vi "Keysight 34461A Measurement Logic.vi"(8 "error in (no error)":errorcluster, 10 "session":refnum<visa-resource-name>, 11 "measurement configuration":T2={"pin_name"="", "measurement_type"=enum."DC Voltage", "auto_range"=FALSE, "manual_range"=0.0, "resolution_digits"=0.0}) -> (0 "error out":errorcluster, 3 "measurement results":T1)   [LabVIEW 2021, in "Keysight 34461A DMM Measurement.lvlib"]
uses:
  Keysight 34461A DMM Measurement.lvlib
  Measurement Results.ctl
  <instrlib>/Agilent 3446X Series/Agilent 3446X Series.lvlib
  <instrlib>/Agilent 3446X Series/Public/Data/Read (Single Point).vi
  Measurement Configuration.ctl
  Keysight 34461A Function.ctl
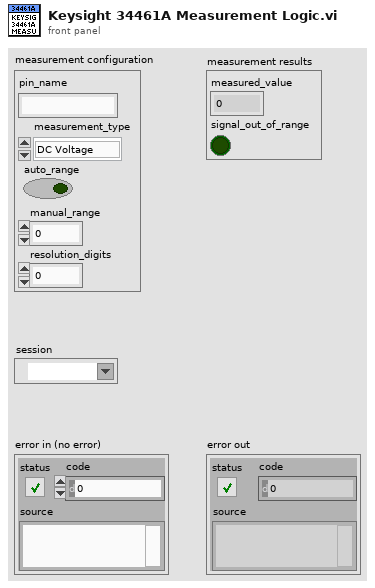
[diagram p1: front panel]
types:
  T1 = typedef "Keysight 34461A DMM Measurement.lvlib/Measurement Results.ctl" = cluster{"measured_value":dbl, "signal_out_of_range":bool}
  T2 = typedef "Keysight 34461A DMM Measurement.lvlib/Measurement Configuration.ctl" = cluster{"pin_name":string, "measurement_type":T3, "auto_range":bool, "manual_range":dbl, "resolution_digits":dbl}
  T3 = typedef "Keysight 34461A DMM Measurement.lvlib/Keysight 34461A Function.ctl" = enum32{"Continuity", "AC Current", "DC Current", "Diode Checking", "Frequency", "4 - Wire Resistance", "Period", "2 - Wire Resistance", "Temperature", "AC Voltage", "DC Voltage", "VDC:VDC Ratio", "Capacitance"}
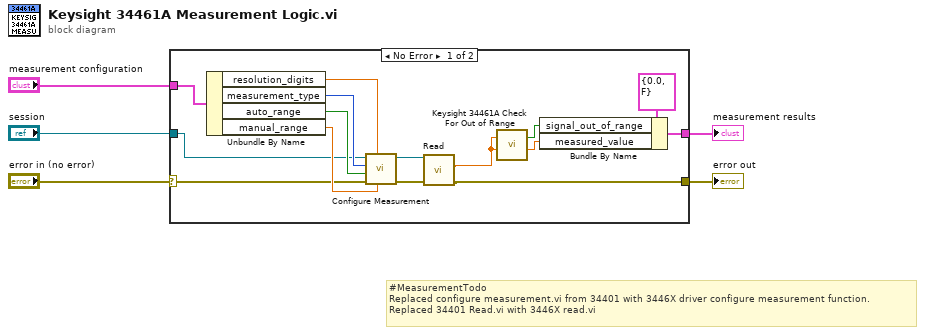
[diagram p0: block diagram]
diagram:
  # "#MeasurementTodo\nReplaced configure measurement.vi from 34401 with 3446X driver configure measurement function.\nReplaced 34401 Read.vi with 3446X read.vi"
  n1 = case shown="No Error" "error in (no error)" {
    selector: "error in (no error)" -> [w11 w20]
    tunnel: "measurement configuration" -> [w19 _]
    tunnel: [w17 _] -> w4
    tunnel: [w6 w20] -> w3
    tunnel: "session" -> [w10 _]
    frame No Error {
      n2 = Unbundle By Name(w19) -> ("resolution_digits"=w15:dbl, "measurement_type"=w14:T3, "auto_range"=w13:bool, "manual_range"=w12:dbl)
      n3 = call <instrlib>:"Configure Measurement.vi"("Manual Range (1)"=w12, "Absolute Resolution (1E-6)"=w15, "error in (no error)"=w11, "Auto Range (T: Enable)"=w13, "Measurement Function (10: Voltage DC)"=w14, "VISA resource name"=w10) -> ("error out"=w9:errorcluster, "VISA resource name out"=w8:refnum<visa-resource-name>)  [unwired: 4 in]
      n4 = call-poly <instrlib>:"Read.vi"("error in (no error)"=w9, "VISA resource name"=w8) -> ("error out"=w6:errorcluster, "Measurement"=w7:dbl)  [unwired: 7 in, 1 out]
      n5 = call "Keysight 34461A Check For Out of Range.vi"("value"=w7) -> ("out of range?"=w16:bool)  [unwired: 2 in]
      n6 = Bundle By Name(cluster=T1 {"measured_value"=0.0, "signal_out_of_range"=FALSE} ("measurement results"), "signal_out_of_range"=w16, "measured_value"=w7) -> (w17:T1)
    }
    frame Error {
    }
  }
  "measurement results" <- w4
  "error out" <- w3
